vi "Dequeue Master and Local.vi"(8 "error in (no error)":errorcluster, 9 "Instrument Name":string, 11 "Message Queues In":T1) -> (0 "error out":errorcluster, 1 "Message Data":variant, 2 "Message":string, 3 "Message Queues out":T1)   [LabVIEW 2014, in "MeasurementControl Message Queue.lvlib"]
doc: "This VI waits for data to arrive at the master queue and it's own UI queue. If items exist in it's UI queue those tasks are done first. Once the UI queue is empty, it looks to see if the message in the master queue is for this particular instrument. If it is, it passes the message along to the UI queue, otherwise it ignores the message and waits for the next one."
uses:
  MeasurementControl Message Queue.lvlib
  All Message Queues.ctl
  Message Cluster.ctl
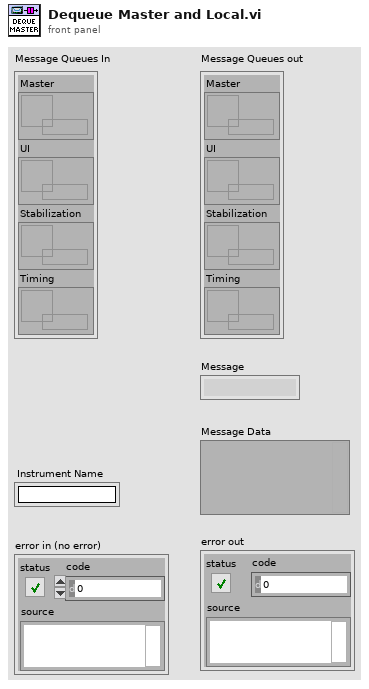
[diagram p1: front panel]
types:
  T1 = typedef "MeasurementControl Message Queue.lvlib/All Message Queues.ctl" = cluster{"Master":refnum<queue>, "UI":refnum<queue>, "Stabilization":refnum<queue>, "Timing":refnum<queue>}
  T2 = typedef "MeasurementControl Message Queue.lvlib/Message Cluster.ctl" = cluster{"Message":string, "Message Data":variant}
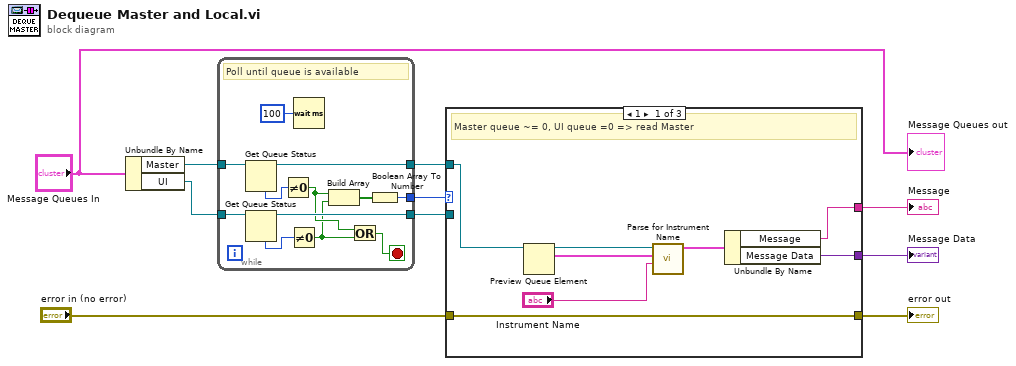
[diagram p0: block diagram]
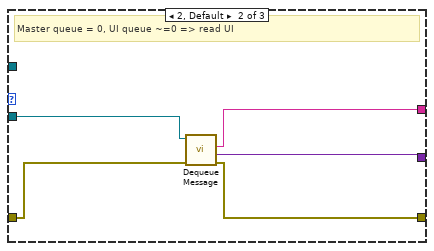
[diagram p2: hidden frame]
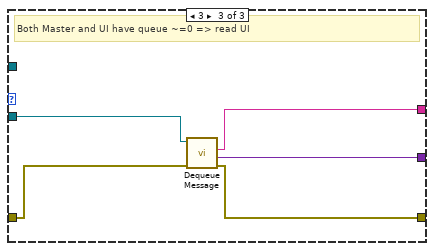
[diagram p3: hidden frame]
diagram:
  n1 = Unbundle By Name("Message Queues In") -> ("Master"=w3:refnum<queue>, "UI"=w2:refnum<queue>)
  n2 = while {
    tunnel: w2 -> [w22]
    tunnel: w3 -> [w19]
    tunnel: [w17] -> w10
    tunnel: [w16] -> w9
    tunnel: [w15] -> w8
    stop <- w13 stop-if-true
    # "Poll until queue is available"
    n3 = Get Queue Status(queue=w19) -> (queue out=w16:refnum<queue>, # elements in queue=w20:i32)  [unwired: 2 in, 6 out]
    n4 = Get Queue Status(queue=w22) -> (queue out=w15:refnum<queue>, # elements in queue=w21:i32)  [unwired: 2 in, 6 out]
    n5 = Not Equal To 0?(x=w20) -> (x != 0?=w12:bool)
    n6 = Not Equal To 0?(x=w21) -> (x != 0?=w11:bool)
    n7 = Wait (ms)(milliseconds to wait=u32 100) -> ()  [unwired: 1 out]
    n8 = Build Array(w12, w11) -> (w18:bool[])
    n9 = Or(x=w12, y=w11) -> (x .or. y?=w13:bool)
    n10 = Boolean Array To Number(Boolean array=w18) -> (number=w17:u32)
  }
  n11 = case shown="1" w10 {
    tunnel: w9 -> [w27 _ _]
    tunnel: w8 -> [_ w31 w36]
    tunnel: "error in (no error)" -> [w28 w32 w40]
    tunnel: [w30 w35 w37] -> w6
    tunnel: [w29 w34 w38] -> w5
    tunnel: [w28 w33 w39] -> w4
    frame 1 {
      # "Master queue ~= 0, UI queue =0 => read Master"
      n12 = Preview Queue Element(queue=w27) -> (queue out=w26:refnum<queue>, element=w24:T2)  [unwired: 2 in, 2 out]
      n13 = call "Parse for Instrument Name.vi"("Instrument Name"="Instrument Name", "Message In"=w24, "Message Queue"=w26) -> ("Message Out"=w23:T2)  [unwired: 8 in]
      n14 = Unbundle By Name(w23) -> ("Message"=w30:string, "Message Data"=w29:variant)
    }
    frame 2, Default {
      # "Master queue = 0, UI queue ~=0 => read UI"
      n15 = call "Dequeue Message.vi"("error in (no error)"=w32, "Message Queue"=w31) -> ("error out"=w33:errorcluster, "Message Data"=w34:variant, "Message"=w35:string)  [unwired: 6 in, 1 out]
    }
    frame 3 {
      # "Both Master and UI have queue ~=0 => read UI"
      n16 = call "Dequeue Message.vi"("error in (no error)"=w40, "Message Queue"=w36) -> ("error out"=w39:errorcluster, "Message Data"=w38:variant, "Message"=w37:string)  [unwired: 6 in, 1 out]
    }
  }
  "error out" <- w4
  "Message Data" <- w5
  "Message" <- w6
  "Message Queues out" <- "Message Queues In"
